vi "Expected Response trigger.vi"(9 "String Buffer in":string, 10 "Force Response":bool, 11 "Expected Response":T1) -> (1 "String Buffer out":string, 2 "Expected Response triggered":bool, 3 "Response":string)   [LabVIEW 2017, in "SSH.lvlib"]
uses:
  SSH.lvlib
  Expected Response String Config.ctl
  Search Start Point.ctl
  String Match Details.ctl
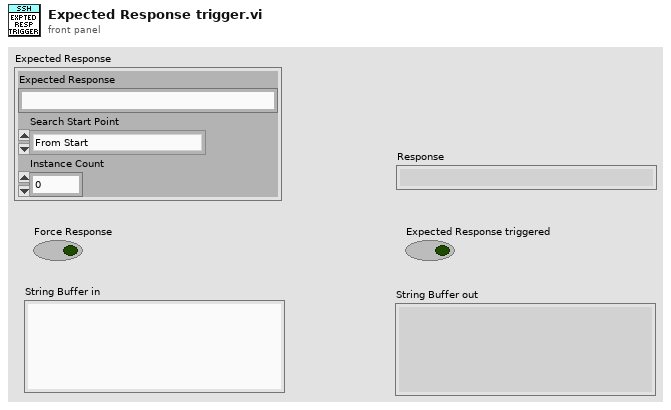
[diagram p1: front panel]
types:
  T1 = typedef "SSH.lvlib/Expected Response String Config.ctl" = cluster{"Expected Response":string, "Search Start Point":T2, "Instance Count":i32}
  T2 = typedef "SSH.lvlib/Search Start Point.ctl" = enum16{"From Start", "From End"}
  T3 = typedef "SSH.lvlib/String Match Details.ctl" = cluster{"Before Match":string, "Match":string, "After Match":string}
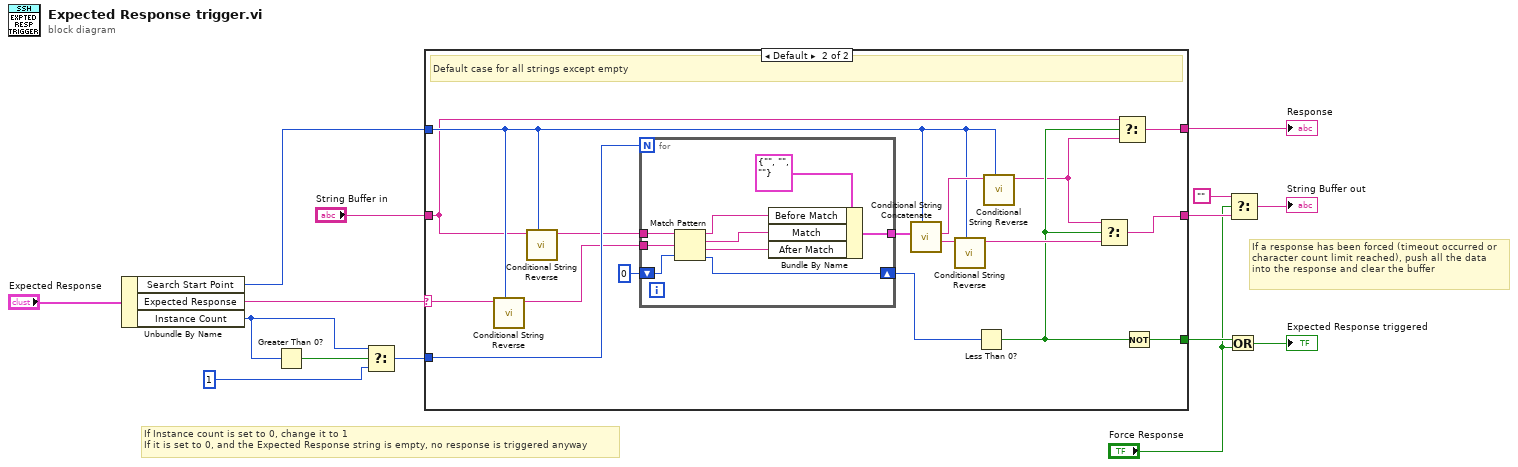
[diagram p0: block diagram]
diagram:
  # "If a response has been forced (timeout occurred or character count limit reached), push all the data into the response and clear the buffer"
  # "If Instance count is set to 0, change it to 1\nIf it is set to 0, and the Expected Response string is empty, no response is triggered anyway"
  n1 = Unbundle By Name("Expected Response") -> ("Search Start Point"=w6:T2, "Expected Response"=w11:string, "Instance Count"=w9:i32)
  n2 = Greater Than 0?(x=w9) -> (x > 0?=w10:bool)
  n3 = Select(t=w9, s=w10, f=1) -> (s? t:f=w8:i32)
  n4 = case shown="Default" w11 {
    selector: w11 -> [_ w32]
    tunnel: [_ w21] -> w15
    tunnel: [w16 w33] -> w4
    tunnel: "String Buffer in" -> [w16 w19]
    tunnel: [w16 w18] -> w13
    tunnel: w6 -> [_ w22]
    tunnel: w8 -> [_ w31]
    frame "" {
      # "Empty string just passes through and doesn't trigger a response"
    }
    frame Default {
      # "Default case for all strings except empty"
      n5 = call "Conditional String Reverse.vi"("Search Start Point"=w22, "String in"=w32) -> ("String out"=w29:string)  [unwired: 9 in]
      n6 = call "Conditional String Reverse.vi"("Search Start Point"=w22, "String in"=w19) -> ("String out"=w28:string)  [unwired: 9 in]
      n7 = for {
        N: w31 -> [_]
        shift-right: [w42] -> w30
        shift-left: 0 ("offset past match") -> [w39]
        tunnel: w29 -> [w41]
        tunnel: w28 -> [w40]
        tunnel: [w35] -> w23
        n8 = Match Pattern(string=w40, regular expression=w41, offset (0)=w39) -> (before substring=w36:string, match substring=w37:string, after substring=w38:string, offset past match=w42:i32)
        n9 = Bundle By Name(cluster=T3 {"Before Match"="", "Match"="", "After Match"=""} ("String Match Details"), "Before Match"=w36, "Match"=w37, "After Match"=w38) -> (w35:T3)
      }
      n10 = call "Conditional String Concatenate.vi"("Search Start Point"=w22, "String Match Details"=w23) -> ("String Buffer out"=w24:string, "Response"=w25:string)  [unwired: 8 in]
      n11 = call "Conditional String Reverse.vi"("Search Start Point"=w22, "String in"=w24) -> ("String out"=w26:string)  [unwired: 9 in]
      n12 = Less Than 0?(x=w30) -> (x < 0?=w20:bool)
      n13 = call "Conditional String Reverse.vi"("Search Start Point"=w22, "String in"=w25) -> ("String out"=w17:string)  [unwired: 9 in]
      n14 = Select(t=w17, s=w20, f=w26) -> (s? t:f=w33:string)
      n15 = Select(t=w19, s=w20, f=w17) -> (s? t:f=w18:string)
      n16 = Not(x=w20) -> (.not. x?=w21:bool)
    }
  }
  "Response" <- w13
  n17 = Or(x=w15, y="Force Response") -> (x .or. y?=→"Expected Response triggered":bool)
  n18 = Select(t="", s="Force Response", f=w4) -> (s? t:f=→"String Buffer out":string)
